vi "main.vi"() -> ()   [LabVIEW 2016]
uses:
  System Status.ctl
  Position Control.ctl
  Manual Operation Control.ctl
  Position Coordinate.ctl
panel:
  out "status":bool
  in  "Test Mode":bool
  in  "Leave HWLS":bool
  in  "Reference":bool
  in  "Reset Motion":bool
  in  "Stop Motion":bool
  in  "Manual Operation Control":T1 {"Speed Override (%)" min=0.0 max=150.0 step=1.0 scale=0.0..150.0; "Rotative"."Step Length" min=0.01 max=100.0 step=0.01; "Rotative"."Speed" min=0.0 max=500.0 step=1.0 scale=0.0..500.0 scale format="%#.0f"; "Linear"."Step Length" min=0.01 max=500.0 step=0.01; "Linear"."Speed" min=0.0 max=500.0 step=1.0 scale=0.0..500.0 scale format="%#.0f"}
  in  "Settings":bool
  in  "Exit":bool
  in  "Initialize":bool
  in  "Auto Run":bool
  in  "Auto Run Control":T2[](array[typedef])
  in  "Rel Position":T3={"Pos X"=0.0, "Position Name"="Rel Move", "Pos Y"=0.0, "Pos Z"=0.0, "Pos A"=0.0, "OK Button"=FALSE, "Normal Move"=FALSE, "Fast Move"=FALSE} {"Pos A" format="%.2f"; "Pos Z" format="%.2f"; "Pos Y" format="%.2f"; "Pos X" format="%.2f"}
  in  "Abs Position":T3={"Pos X"=0.0, "Position Name"="Abs Move", "Pos Y"=0.0, "Pos Z"=0.0, "Pos A"=0.0, "OK Button"=FALSE, "Normal Move"=FALSE, "Fast Move"=FALSE} {"Pos A" format="%.2f"; "Pos Z" format="%.2f"; "Pos Y" format="%.2f"; "Pos X" format="%.2f"}
  out "System Status":T4 {"Axis A"."Position" format="%.2f"; "Axis Z"."Position" format="%.2f"; "Axis Y"."Position" format="%.2f"; "Rotativ Speed" format="%#_6f"; "Linear Speed" format="%#.2f"; "Axis X"."Position" format="%.2f"}
  out "Error Information":string
  in  "MotionLibrary Path":path=path "C:/Program Files (x86)/National Instruments/LabVIEW 2016/user.lib/iselmotion/CNCAPI/CtrlDll/Dummy/mctlDummy.dll"
  out "Motor hModule":i32
  in  "MotionIni File In":path=path "C:/Program Files (x86)/National Instruments/LabVIEW 2016/user.lib/iselmotion/CNCAPI/CtrlDll/Dummy/MctlDummy.INI"
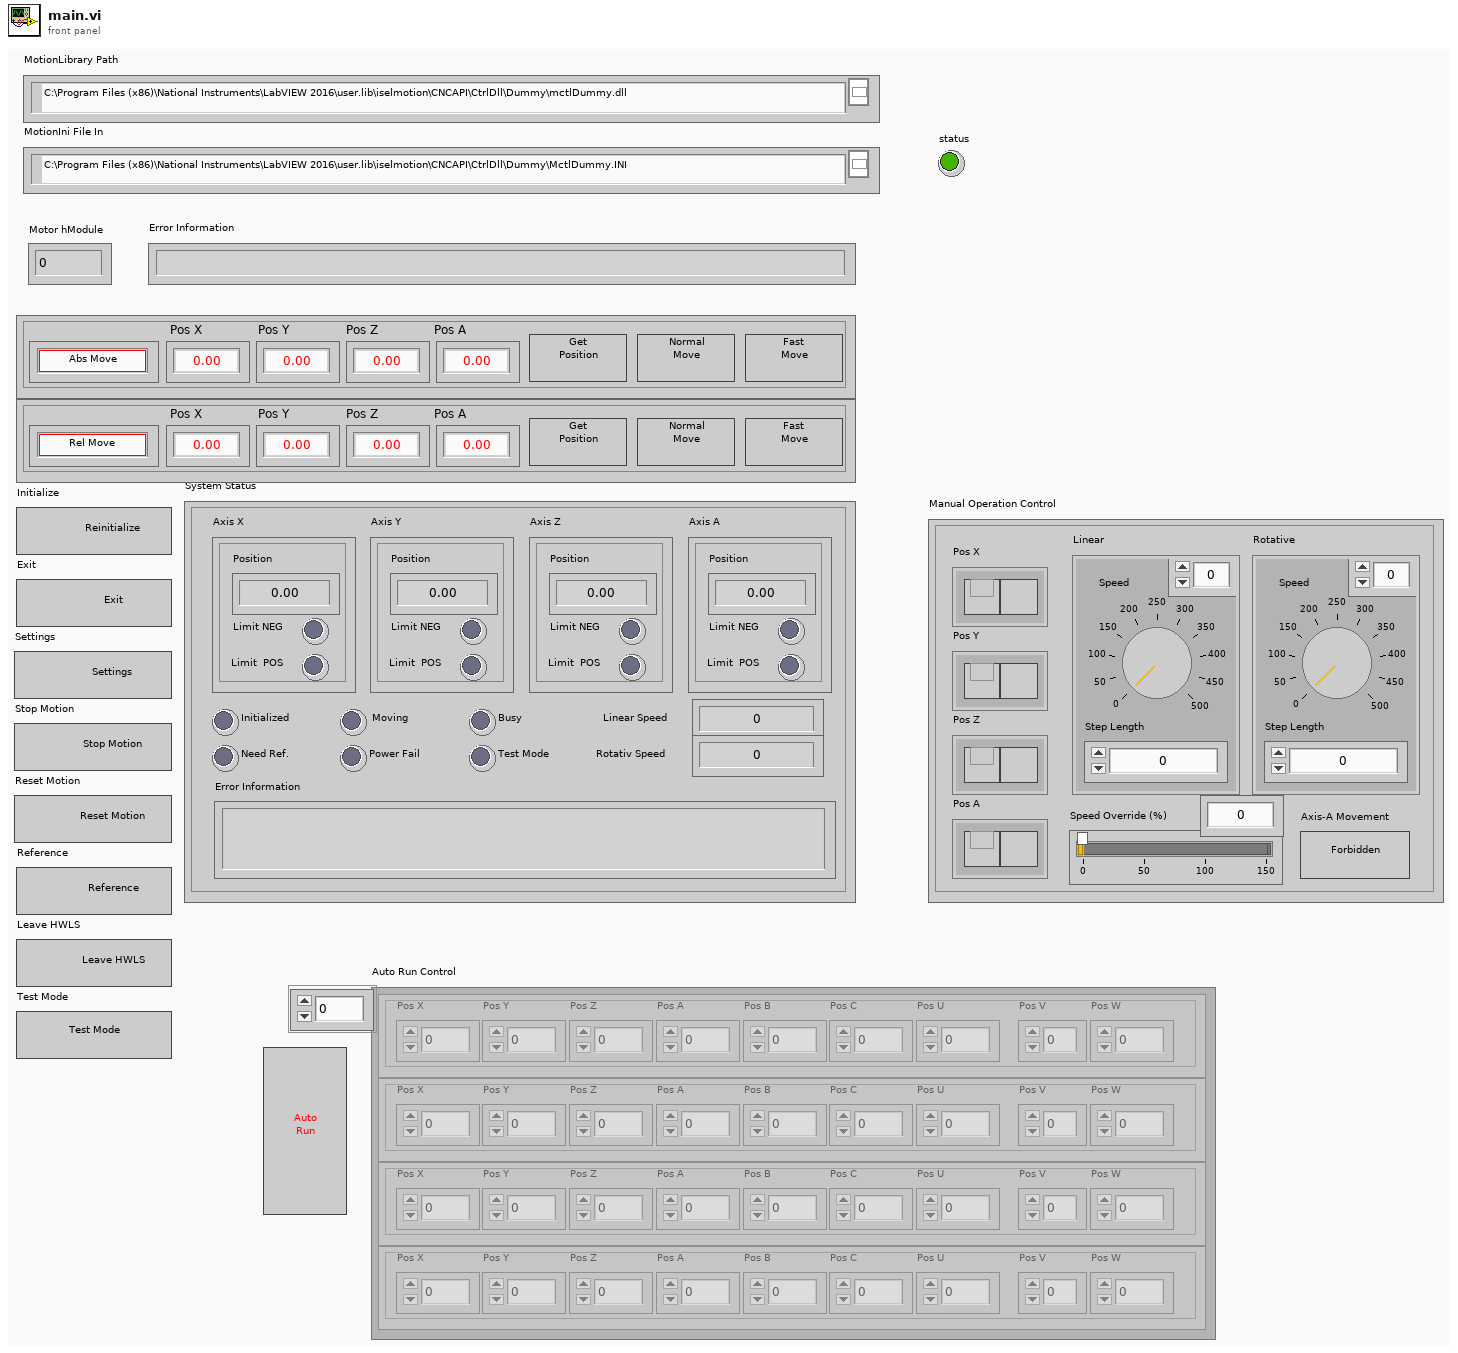
[diagram p1: front panel]
types:
  T1 = typedef "Manual Operation Control.ctl" = cluster{"Pos X":cluster{"Plus":bool, "Minus":bool}, "Pos Y":cluster{"Plus":bool, "Minus":bool}, "Pos Z":cluster{"Plus":bool, "Minus":bool}, "Pos A":cluster{"Plus":bool, "Minus":bool}, "Linear":cluster{"Speed":dbl, "Step Length":dbl}, "Rotative":cluster{"Speed":dbl, "Step Length":dbl}, "Speed Override (%)":dbl, "Axis-A Movement":bool}
  T2 = typedef "Position Coordinate.ctl" = cluster{"Pos X":dbl, "Pos Y":dbl, "Pos Z":dbl, "Pos A":dbl, "Pos B":dbl, "Pos C":dbl, "Pos U":dbl, "Pos V":dbl, "Pos W":dbl}
  T3 = typedef "Position Control.ctl" = cluster{"Pos X":dbl, "Position Name":string, "Pos Y":dbl, "Pos Z":dbl, "Pos A":dbl, "OK Button":bool, "Normal Move":bool, "Fast Move":bool}
  T4 = typedef "System Status.ctl" = cluster{"Axis X":cluster{"Position":dbl, "Limit NEG":bool, "Limit  POS":bool}, "Axis Y":cluster{"Position":dbl, "Limit NEG":bool, "Limit  POS":bool}, "Axis Z":cluster{"Position":dbl, "Limit NEG":bool, "Limit  POS":bool}, "Axis A":cluster{"Position":dbl, "Limit NEG":bool, "Limit  POS":bool}, "Initialized":bool, " Moving":bool, "Busy":bool, "Need Ref.":bool, "Power Fail":bool, "Test Mode":bool, "Linear Speed":dbl, "Rotativ Speed":dbl, "Error Information":string}
  T5 = enum16{"open", "replace", "create", "open or create", "replace or create", "replace or create with confirmation"}
  T6 = enum8{"Enabled", "Disabled", "Disabled and Grayed Out"}
  T7 = cluster{"PosX":i32, "PosY":i32, "PosZ":i32, "PosA":i32, "PosB":i32, "PosC":i32, "PosU":i32, "PosV":i32, "PosW":i32}
  T8 = cluster{"MotionLibrary Path":path, "MotionIni File In":path}
  T9 = cluster{"Common":cluster{"INMOTION":bool, "INSTOPMODE":bool, "INTEACHMODE":bool, "INTESTMODE":bool, "CURRENTOFF":bool, "INPATHMOTION":bool, "ISMOVING":bool, "PATHSTARTED":bool, "NEEDREFERENCERUN":bool, "BREAKERROR":bool, "HWLSACTIVE":bool, "SWLSACTIVE":bool, "HWLSDURINGMOTION":bool, "AFTERRUNERROR":bool, "LOADPATHDATAERROR":bool, "KEYSWITCHERROR":bool, "KEYSWDURINGMOTION":bool, "POWER_FAIL":bool, "SC_FAIL":bool, "HARDWARE_FAIL":bool, "COMMUNICATION_FAIL":bool}, "HWLSNeg":cluster{"HWLS_X_NEG":bool, "HWLS_Y_NEG":bool, "HWLS_Z_NEG":bool, "HWLS_A_NEG":bool, "HWLS_B_NEG":bool, "HWLS_C_NEG":bool, "HWLS_U_NEG":bool, "HWLS_V_NEG":bool, "HWLS_W_NEG":bool}, "HWLSPos":cluster{"HWLS_X_POS":bool, "HWLS_Y_POS":bool, "HWLS_Z_POS":bool, "HWLS_A_POS":bool, "HWLS_B_POS":bool, "HWLS_C_POS":bool, "HWLS_U_POS":bool, "HWLS_V_POS":bool, "HWLS_W_POS":bool}, "SWLSNeg":cluster{"SWLS_X_NEG":bool, "SWLS_Y_NEG":bool, "SWLS_Z_NEG":bool, "SWLS_A_NEG":bool, "SWLS_B_NEG":bool, "SWLS_C_NEG":bool, "SWLS_U_NEG":bool, "SWLS_V_NEG":bool, "SWLS_W_NEG":bool}, "SWLSPos":cluster{"SWLS_X_POS":bool, "SWLS_Y_POS":bool, "SWLS_Z_POS":bool, "SWLS_A_POS":bool, "SWLS_B_POS":bool, "SWLS_C_POS":bool, "SWLS_U_POS":bool, "SWLS_V_POS":bool, "SWLS_W_POS":bool}, "Extended":cluster{"ISBUSY":bool, "DISABLED":bool, "ISINITIALIZED":bool, "READY":bool, "DRILLCYCLEACTIVE":bool, "CTRLSPECERROR":bool}, "Additional flags":cluster{"InMotion":bool, "InStopMode":bool, "InTeachMode":bool, "InTestMode":bool, "CurrentOff":bool, "InPathMotion":bool, "IsMoving":bool, "NeedReferenceRun":bool, "BreakError":bool, "HWLSActive":bool, "SWLSActive":bool, "HWLSDuringMotion":bool, "AfterRunError":bool, "PowerFail":bool, "SCFail":bool, "IsBusy":bool, "Initialized":bool, "Disabled":bool, "HardwareFail":bool, "CommunicationFail":bool, "DrillCycleActive":bool, "CtrlSpecError":bool, "PathStarted":bool}}
  T10 = cluster{"PosX":dbl, "PosY":dbl, "PosZ":dbl, "PosA":dbl, "PosB":dbl, "PosC":dbl, "PosU":dbl, "PosV":dbl, "PosW":dbl}
  T11 = cluster{"PosX":dbl, "HWLS_X_NEG":bool, "HWLS_X_POS":bool}
  T12 = cluster{"PosY":dbl, "HWLS_Y_NEG":bool, "HWLS_Y_POS":bool}
  T13 = cluster{"PosZ":dbl, "HWLS_Z_NEG":bool, "HWLS_Z_POS":bool}
  T14 = cluster{dbl, "HWLS_A_NEG":bool, "HWLS_A_POS":bool}
  T15 = cluster{"LiNormVel":i32, "DrNormVel":i32, "LiFastVel":i32, "DrFastVel":i32, "LiTeachVel":i32, "DrTeachVel":i32, "LiActVel":i32, "DrActVel":i32}
  T16 = cluster{"LiNormVel":dbl, "DrNormVel":dbl, "LiFastVel":dbl, "DrFastVel":dbl, "LiTeachVel":dbl, "DrTeachVel":dbl, "LiActVel":dbl, "DrActVel":dbl}
  T17 = cluster{"Ability":cluster{"LINEAR":bool, "CIRCLE":bool, "HELIX":bool, "SPLINE":bool, "BEZIER":bool, "PRECALC":bool, "ONLINE":bool}, "NumAxis":u32, "AxisConfig":cluster{"AxisConfig 0":cluster{"Type":cluster{"LINEAR":bool, "ROT":bool}, "In Use":bool, "ID":u32, "RangeMin":u32, "RangeMax":u32}, "AxisConfig 1":cluster{"Type":cluster{"LINEAR":bool, "ROT":bool}, "In Use":bool, "ID":u32, "RangeMin":u32, "RangeMax":u32}, "AxisConfig 2":cluster{"Type":cluster{"LINEAR":bool, "ROT":bool}, "In Use":bool, "ID":u32, "RangeMin":u32, "RangeMax":u32}, "AxisConfig 3":cluster{"Type":cluster{"LINEAR":bool, "ROT":bool}, "In Use":bool, "ID":u32, "RangeMin":u32, "RangeMax":u32}, "AxisConfig 4":cluster{"Type":cluster{"LINEAR":bool, "ROT":bool}, "In Use":bool, "ID":u32, "RangeMin":u32, "RangeMax":u32}, "AxisConfig 5":cluster{"Type":cluster{"LINEAR":bool, "ROT":bool}, "In Use":bool, "ID":u32, "RangeMin":u32, "RangeMax":u32}, "AxisConfig 6":cluster{"Type":cluster{"LINEAR":bool, "ROT":bool}, "In Use":bool, "ID":u32, "RangeMin":u32, "RangeMax":u32}, "AxisConfig 7":cluster{"Type":cluster{"LINEAR":bool, "ROT":bool}, "In Use":bool, "ID":u32, "RangeMin":u32, "RangeMax":u32}, "AxisConfig 8":cluster{"Type":cluster{"LINEAR":bool, "ROT":bool}, "In Use":bool, "ID":u32, "RangeMin":u32, "RangeMax":u32}}}
  T18 = cluster{"In Use":bool, "In Use":bool, "In Use":bool, "In Use":bool, "In Use":bool, "In Use":bool, "In Use":bool, "In Use":bool, "In Use":bool}
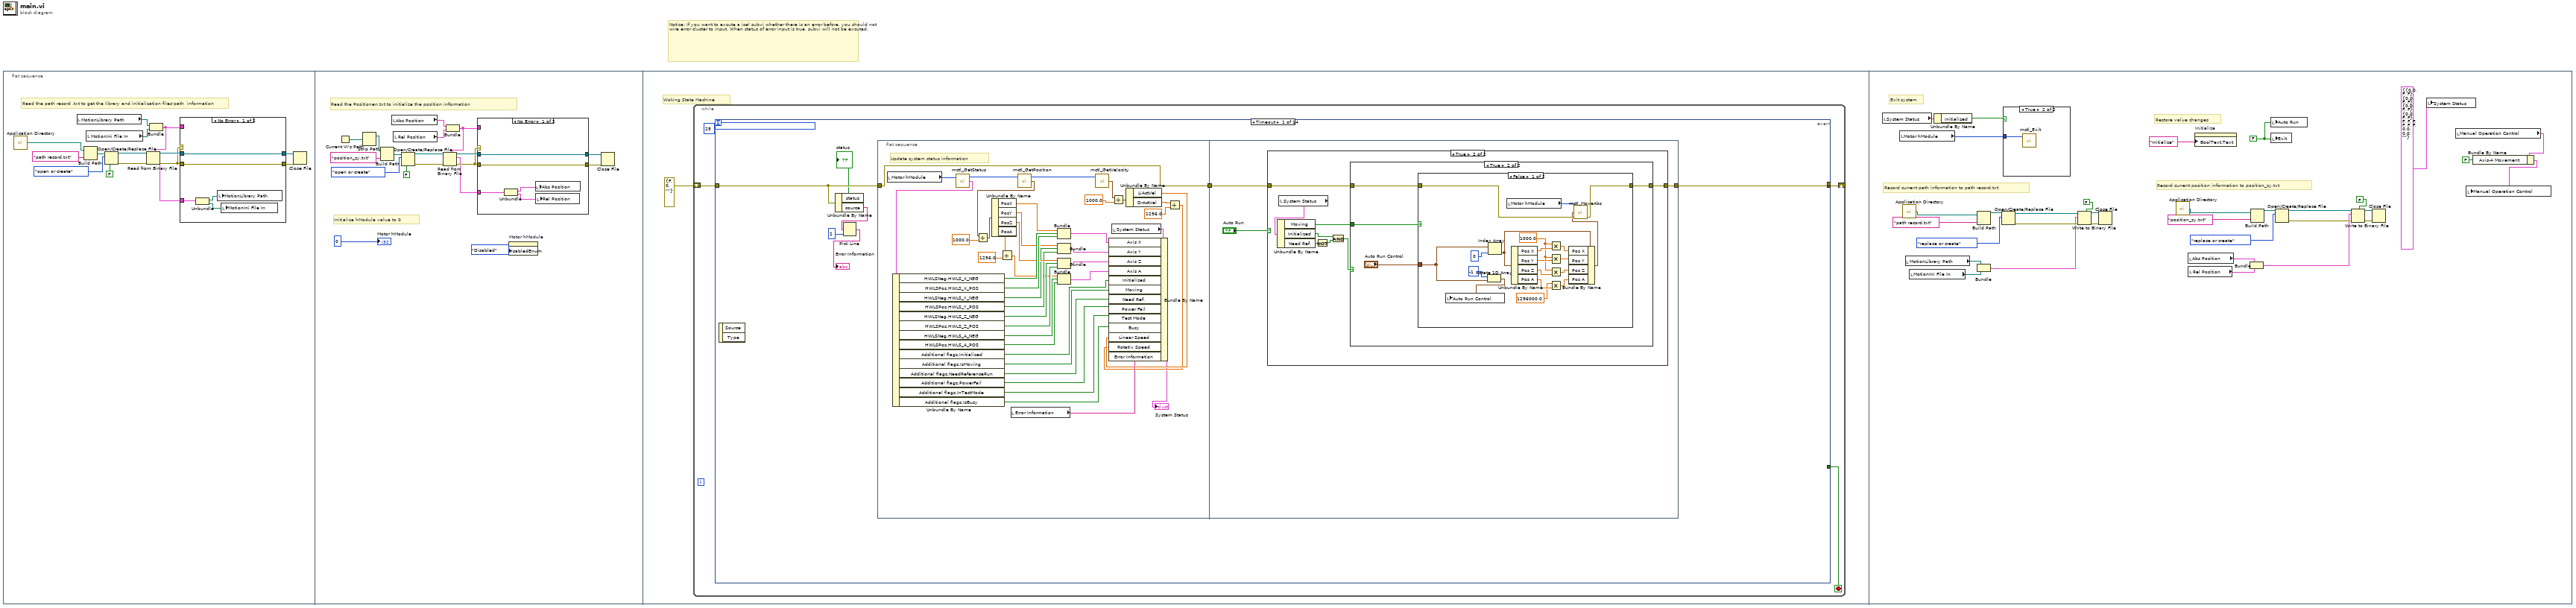
[diagram p0: block diagram]
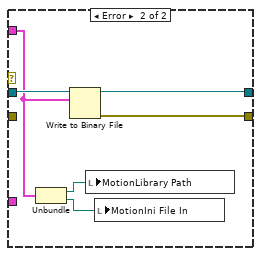
[diagram p2: hidden frame]
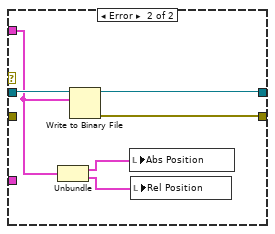
[diagram p3: hidden frame]
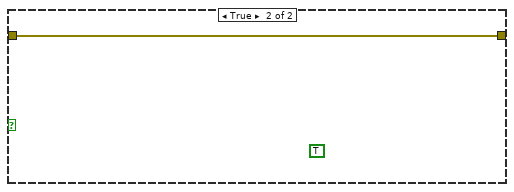
[diagram p6: hidden frame]
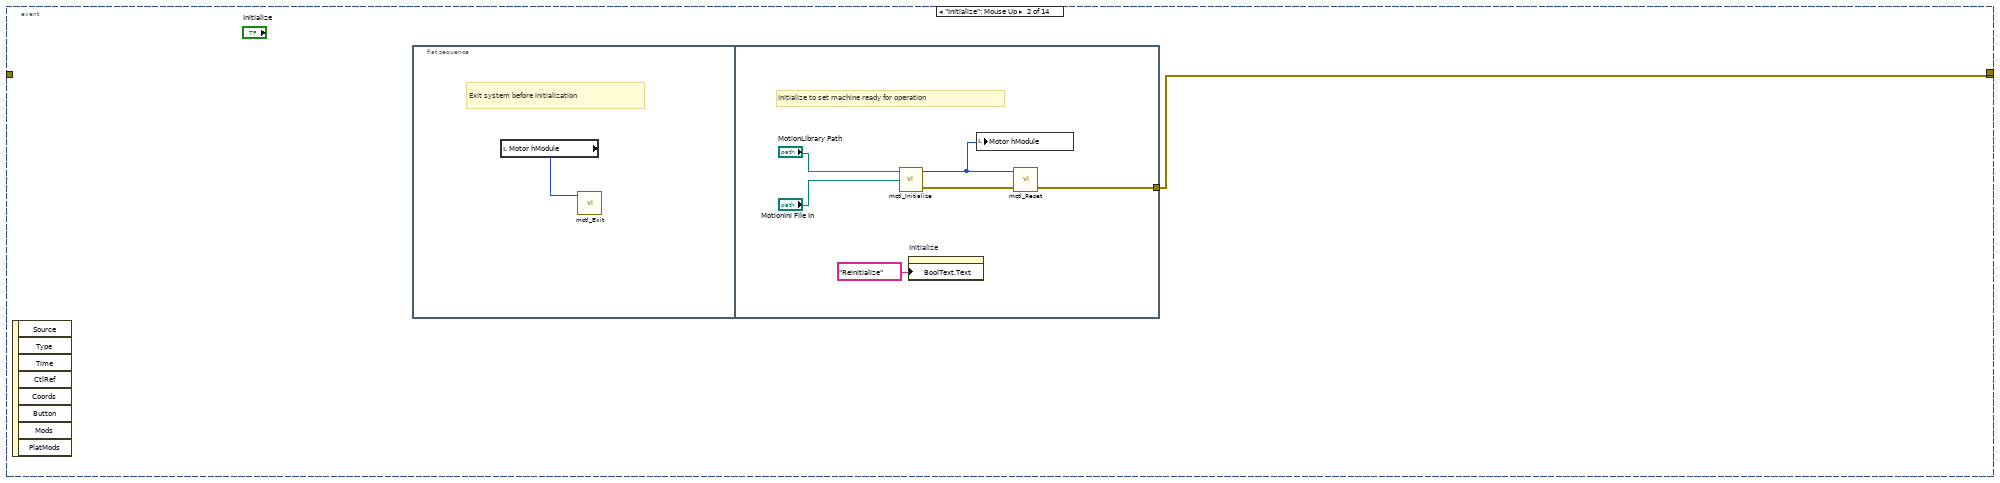
[diagram p7: hidden frame]
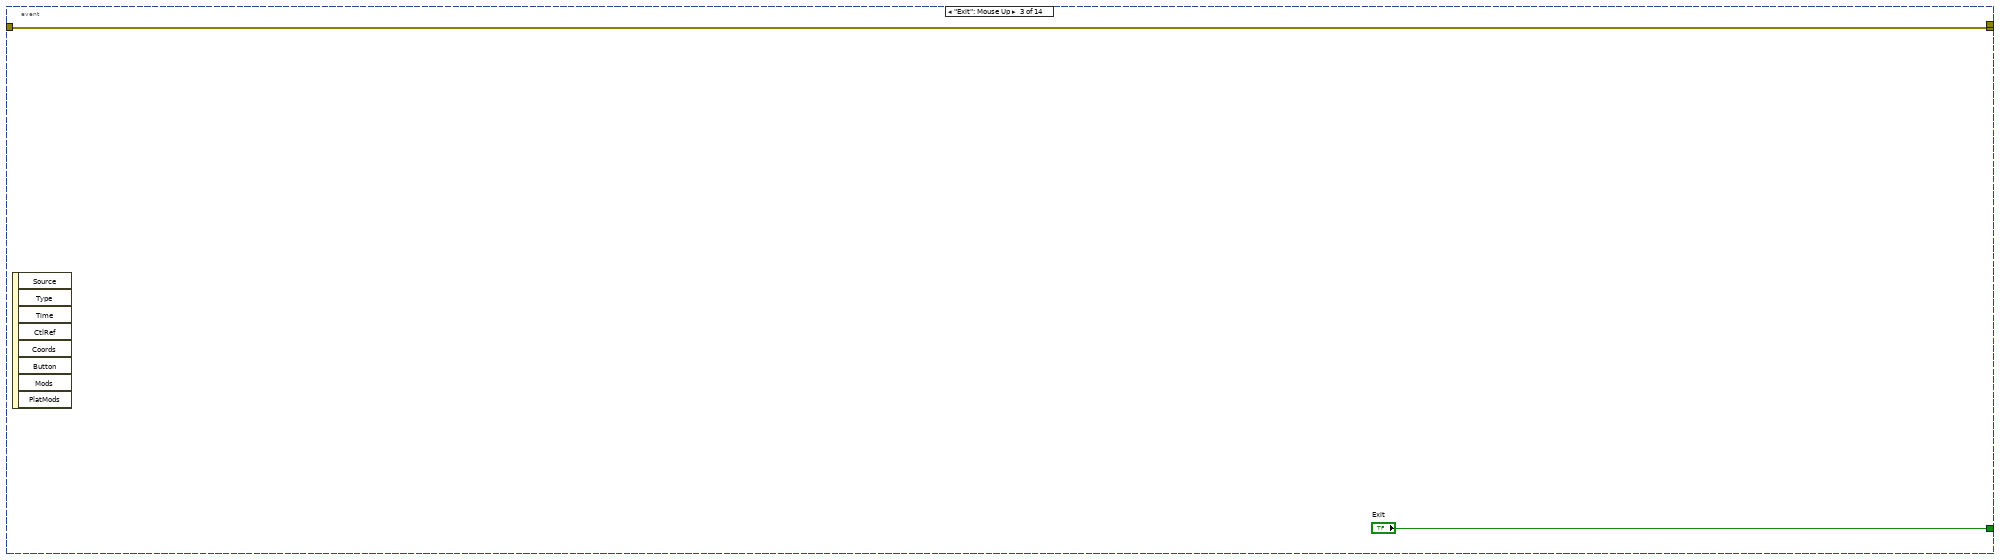
[diagram p8: hidden frame]
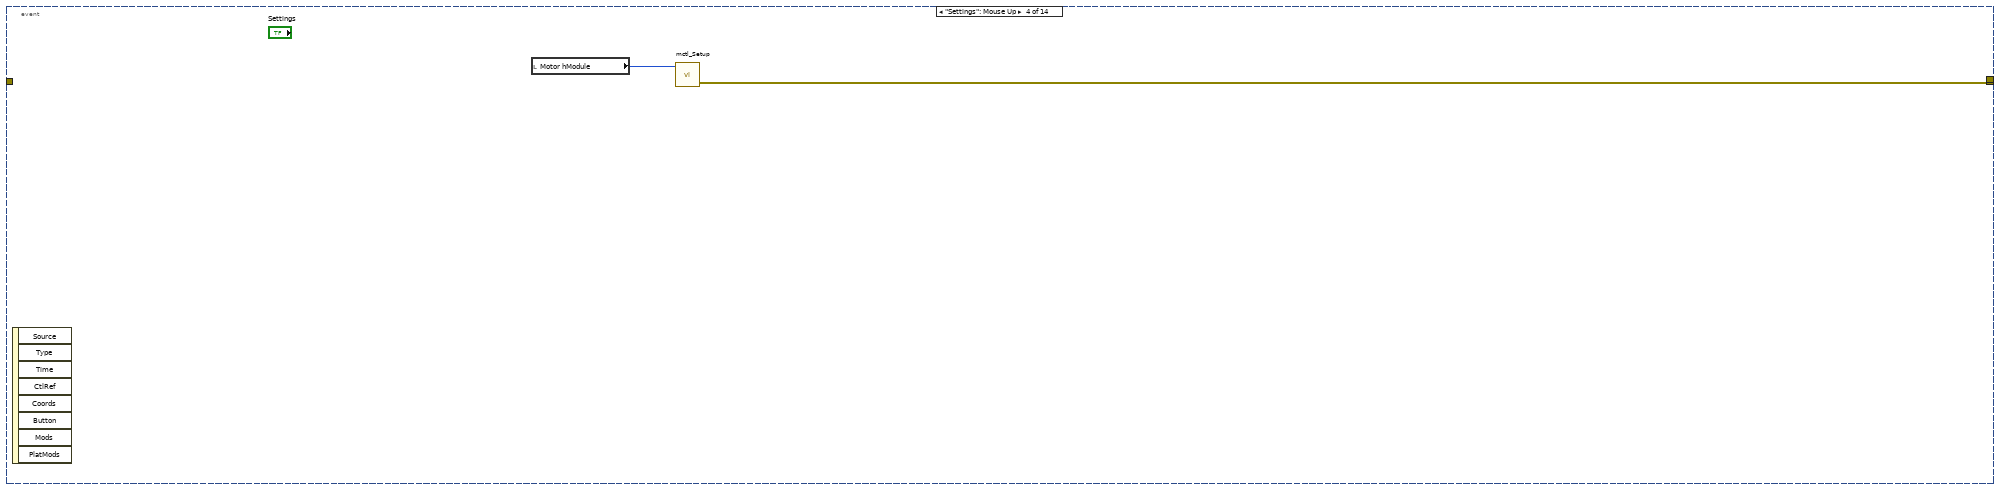
[diagram p9: hidden frame]
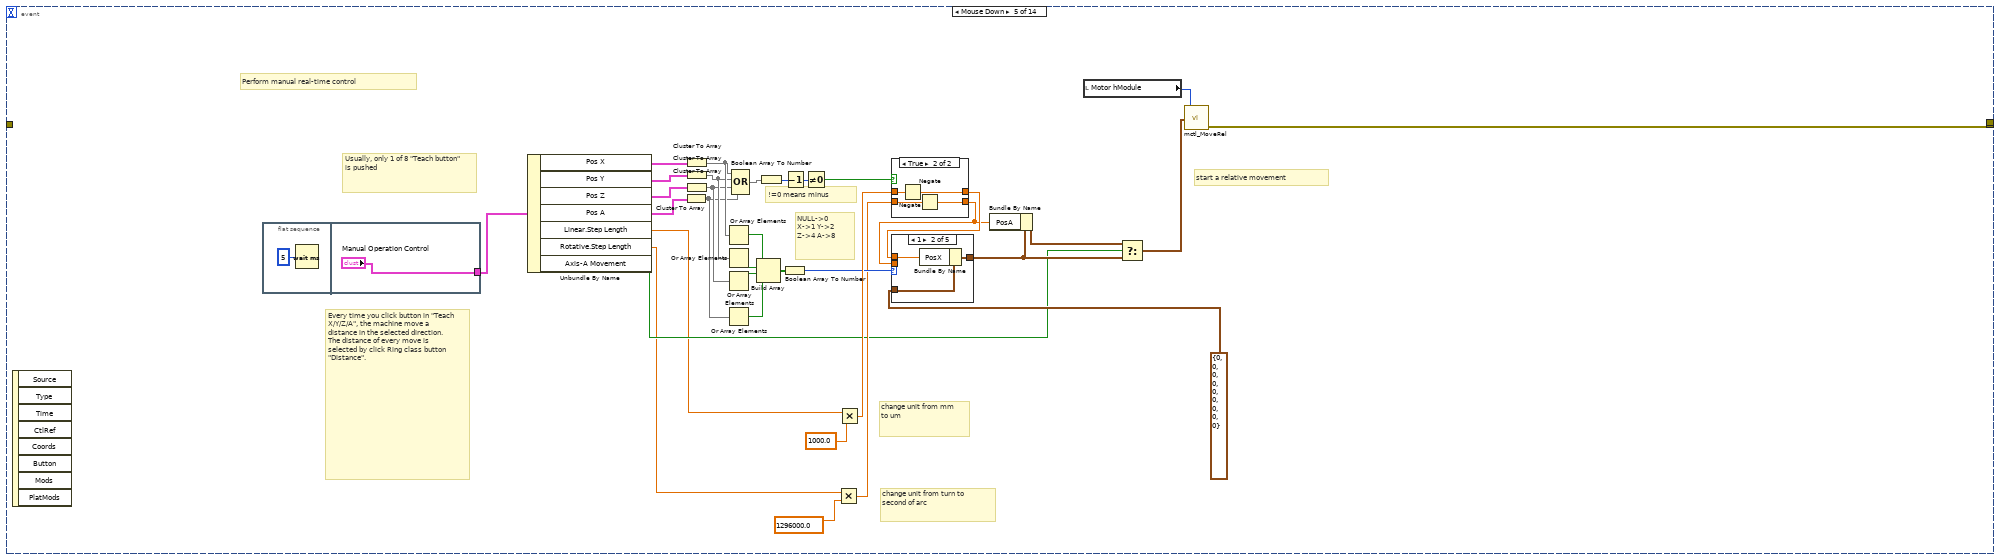
[diagram p10: hidden frame]
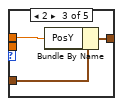
[diagram p12: hidden frame]
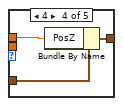
[diagram p13: hidden frame]
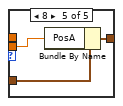
[diagram p14: hidden frame]
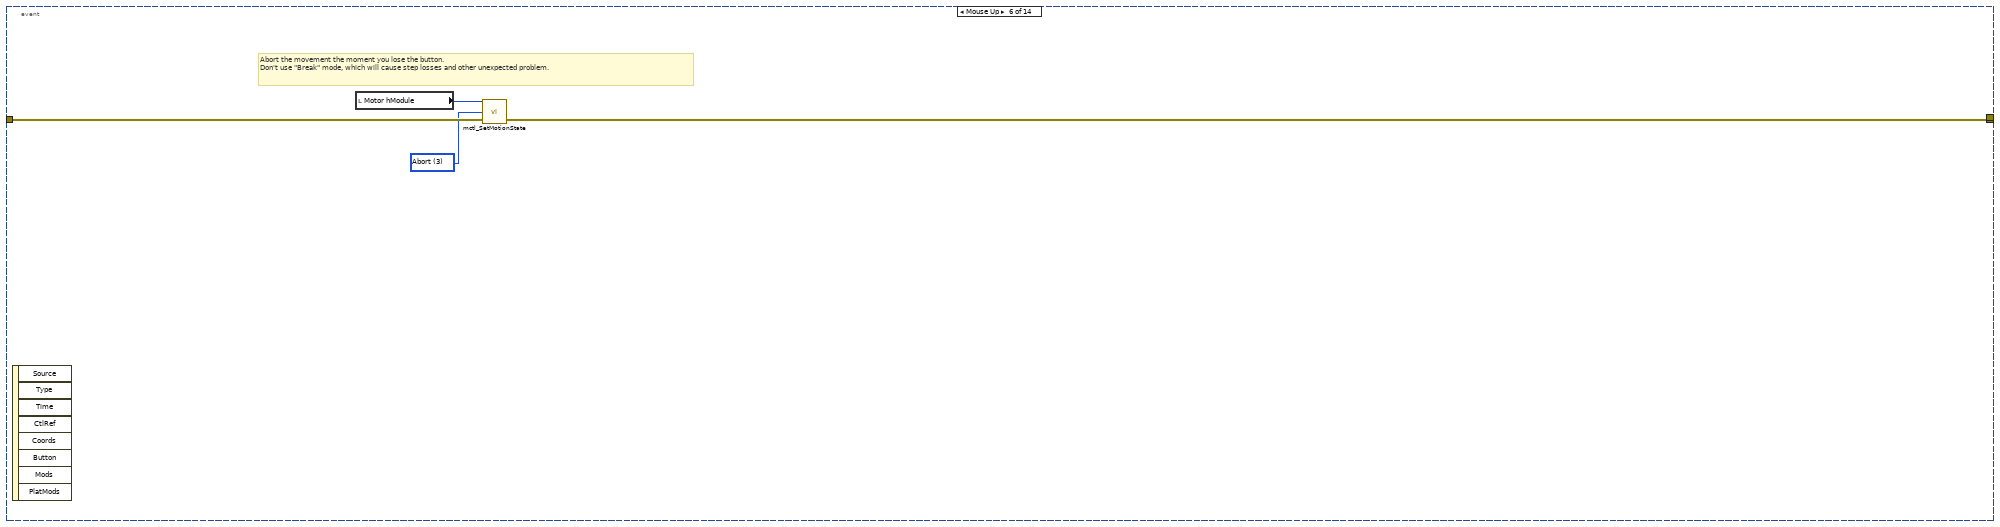
[diagram p16: hidden frame]
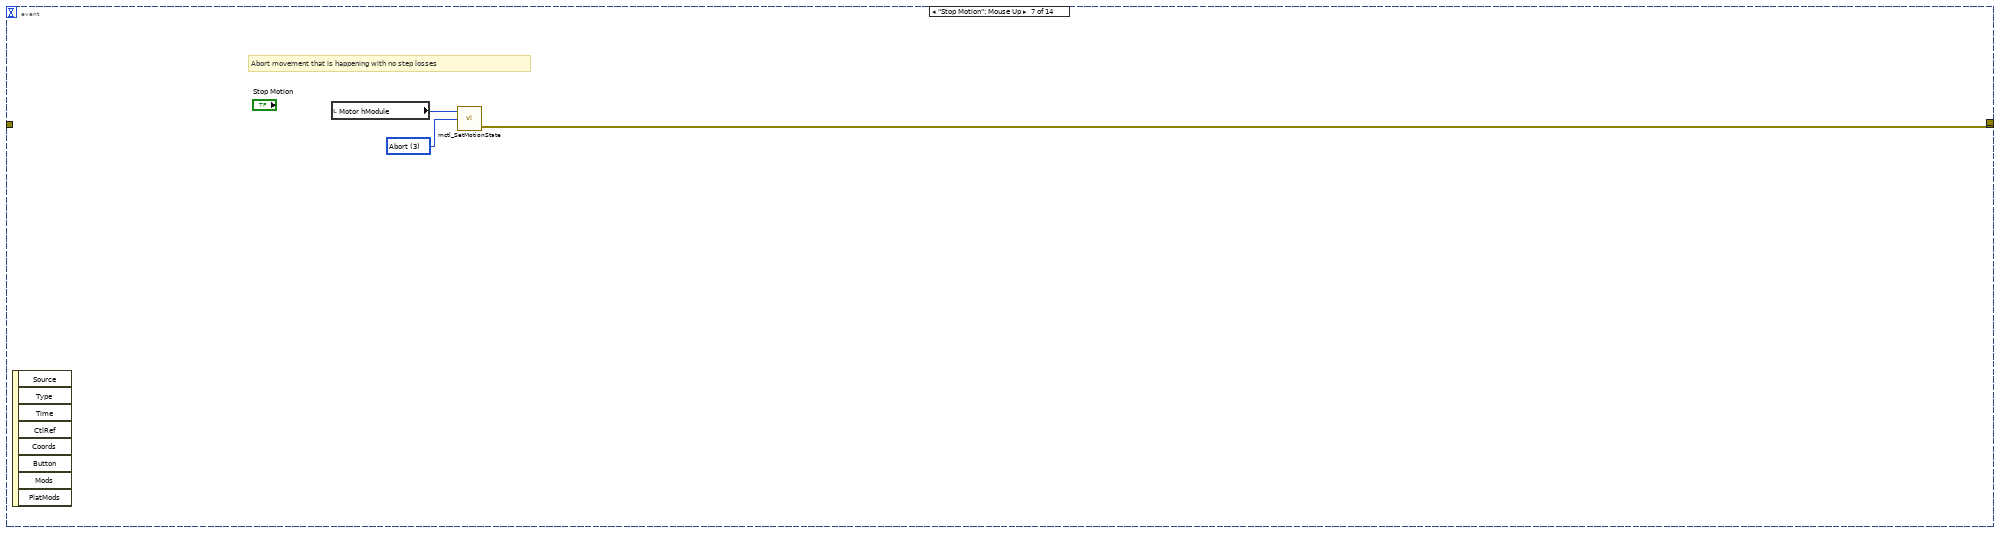
[diagram p17: hidden frame]
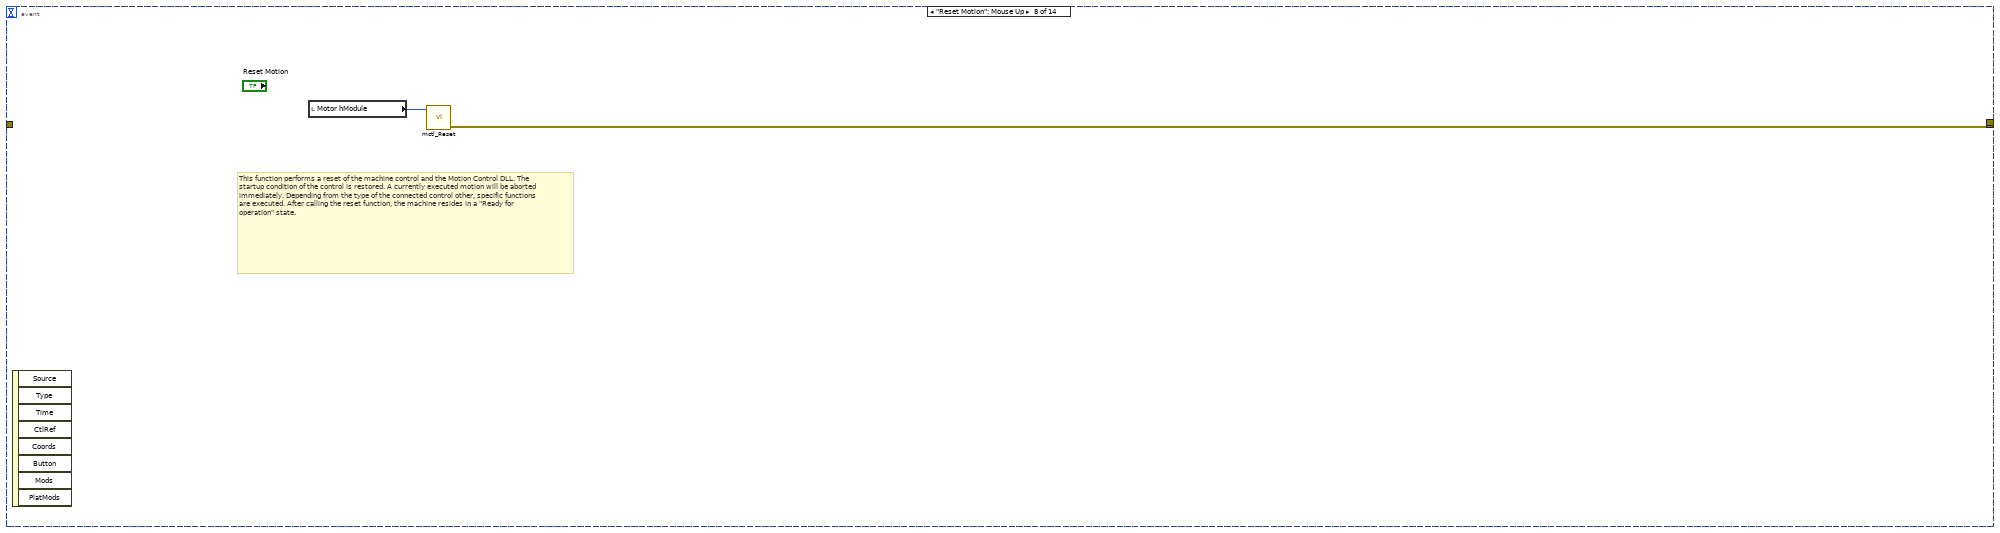
[diagram p18: hidden frame]
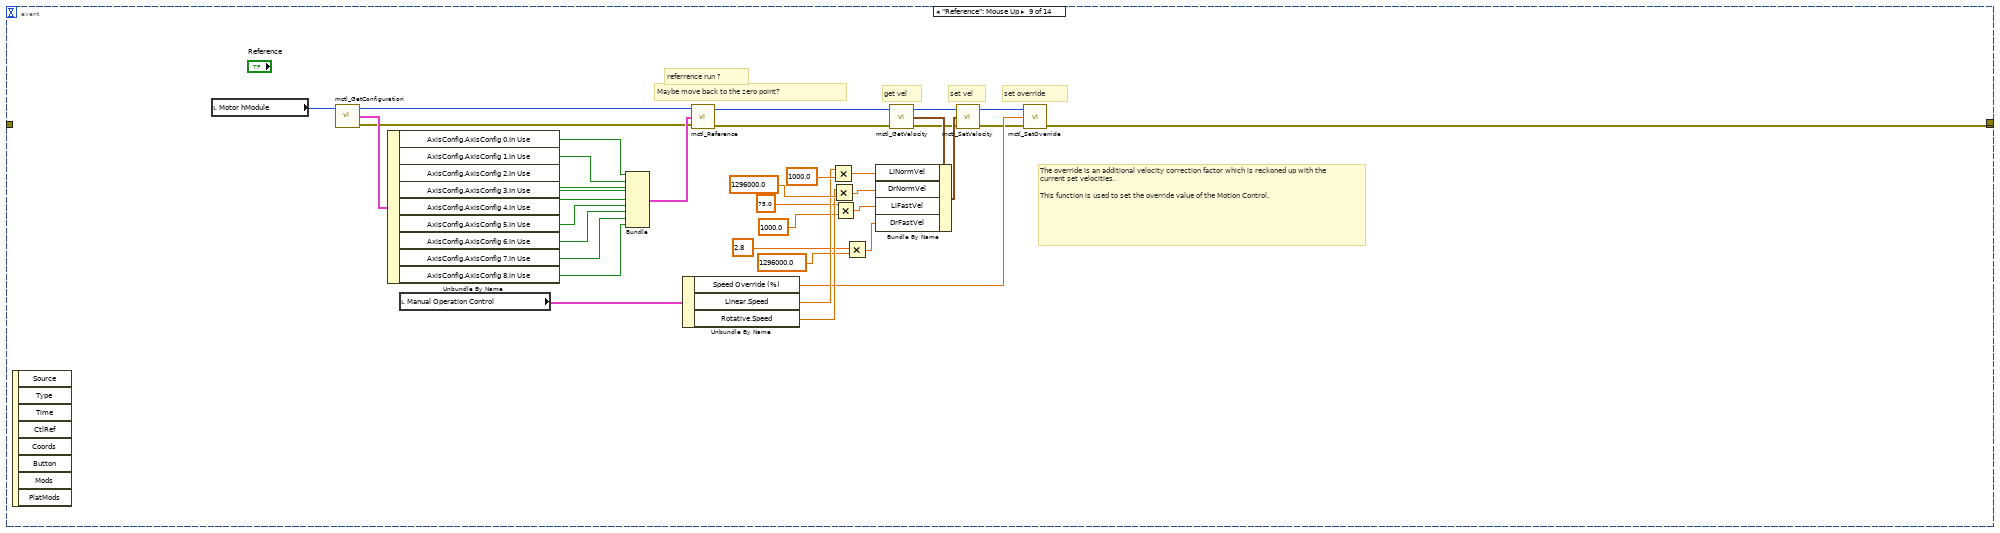
[diagram p19: hidden frame]
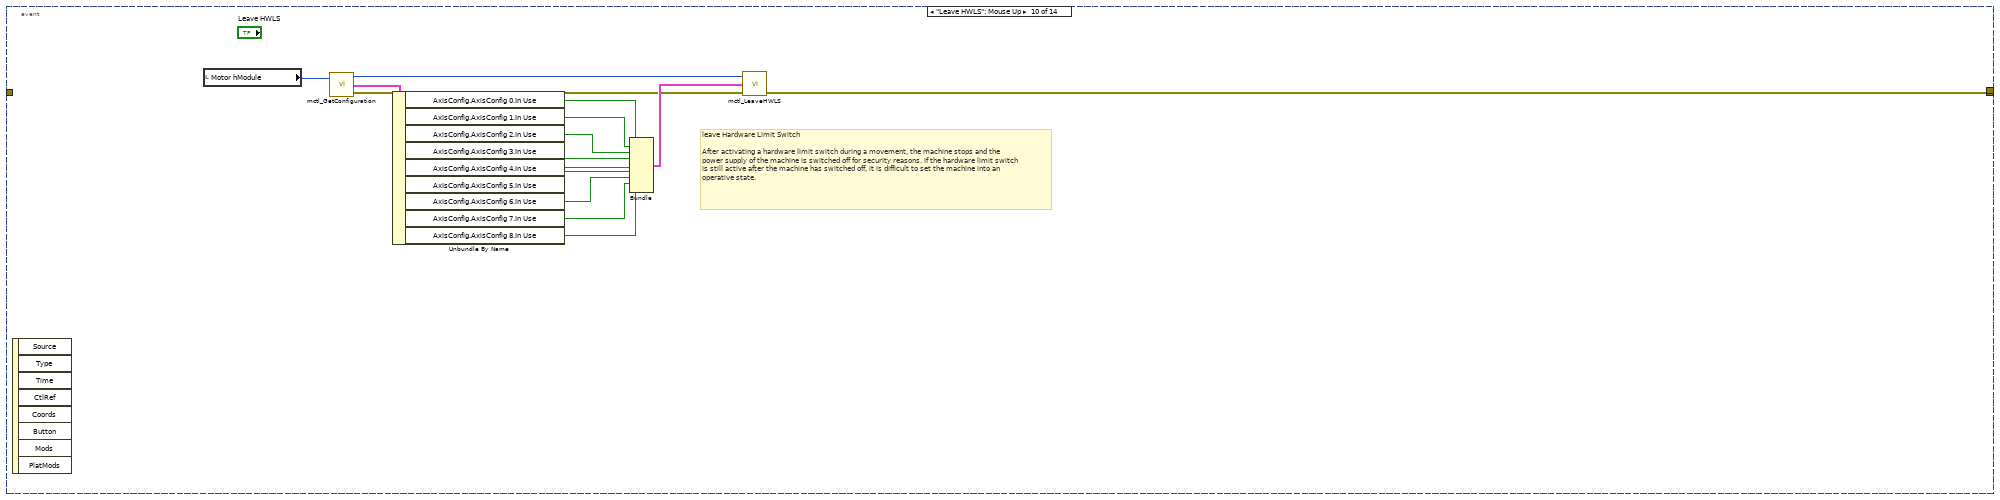
[diagram p20: hidden frame]
diagram:
  # "Notice: If you want to excute a isel subvi whether there is an error before, you should not wire error cluster to input. When status of error input is true, subvi will not be excuted."
  n1 = flat-sequence {
    frame #0 {
      # "Read the path record .txt to get the library and initialization files'path  information"
      n2 = call <vilib>:"Application Directory.vi"() -> ("Application Directory"=w2:path)
      n3 = local read "MotionLibrary Path"() -> (w10:path)
      n4 = Build Path(base path=w2, name or relative path="path record.txt") -> (appended path=w13:path)
      n5 = local read "MotionIni File In"() -> (w11:path)
      n6 = Open/Create/Replace File(file path (use dialog)=w13, operation (0:open)=T5."open or create", disable buffering (F)=FALSE ("advisory dialog? (display:T)")) -> (refnum out=w15:refnum<file>, error out=w12:errorcluster)  [unwired: 3 in, 1 out]
      n7 = Bundle("MotionLibrary Path"=w10, "MotionIni File In"=w11) -> (w3:T8)  [unwired: 1 in]
      n8 = Read from Binary File(5:w3, 8:w12, 11:w15) -> (0:w4:errorcluster, 2:w1:T8, 3:w7:refnum<file>)  [unwired: 3 in, 1 out]
      n9 = case shown="No Error" w4 {
        tunnel: w7 -> [w20 w26]
        tunnel: [w20 w24] -> w6
        tunnel: [w19 w25] -> w5
        tunnel: w4 -> [w19 _]
        tunnel: w3 -> [_ w23]
        tunnel: w1 -> [w18 _]
        frame No Error {
          n10 = Unbundle(w18) -> ("MotionLibrary Path"=w17:path, "MotionIni File In"=w16:path)
          n11 = local write "MotionLibrary Path"(w17) -> ()
          n12 = local write "MotionIni File In"(w16) -> ()
        }
        frame Error {
          n13 = Unbundle(w23) -> ("MotionLibrary Path"=w22:path, "MotionIni File In"=w21:path)
          n14 = Write to Binary File(file (use dialog)=w26, data=w23) -> (refnum out=w24:refnum<file>, error out=w25:errorcluster)  [unwired: 4 in, 1 out]
          n15 = local write "MotionLibrary Path"(w22) -> ()
          n16 = local write "MotionIni File In"(w21) -> ()
        }
      }
      n17 = Close File(refnum=w6, error in=w5) -> ()  [unwired: 2 out]
    }
    frame #1 {
      # "Initialize hModule value to 0"
      # "Read the Positionen.txt to initialize the position information"
      n18 = Current VI's Path() -> (path=w30:path)
      n19 = Strip Path(path=w30) -> (stripped path=w43:path)  [unwired: 1 out]
      n20 = Build Path(base path=w43, name or relative path="position_zy.txt") -> (appended path=w41:path)
      n21 = local read "Abs Position"() -> (w38:T3)
      n22 = local read "Rel Position"() -> (w39:T3)
      n23 = Open/Create/Replace File(file path (use dialog)=w41, operation (0:open)=T5."open or create", disable buffering (F)=FALSE ("advisory dialog? (display:T)")) -> (refnum out=w44:refnum<file>, error out=w40:errorcluster)  [unwired: 3 in, 1 out]
      n24 = Bundle("Abs Position"=w38, "Rel Position"=w39) -> (w31:cluster{"Abs Position":T3, "Rel Position":T3})  [unwired: 1 in]
      n25 = Read from Binary File(5:w31, 8:w40, 11:w44) -> (0:w32:errorcluster, 2:w28:cluster{"Abs Position":T3, "Rel Position":T3}, 3:w35:refnum<file>)  [unwired: 3 in, 1 out]
      n26 = case shown="No Error" w32 {
        tunnel: w35 -> [w49 w55]
        tunnel: [w49 w53] -> w34
        tunnel: [w48 w54] -> w33
        tunnel: w32 -> [w48 _]
        tunnel: w31 -> [_ w52]
        tunnel: w28 -> [w47 _]
        frame No Error {
          n27 = Unbundle(w47) -> ("Abs Position"=w46:T3, "Rel Position"=w45:T3)
          n28 = local write "Abs Position"(w46) -> ()
          n29 = local write "Rel Position"(w45) -> ()
        }
        frame Error {
          n30 = Unbundle(w52) -> ("Abs Position"=w51:T3, "Rel Position"=w50:T3)
          n31 = Write to Binary File(file (use dialog)=w55, data=w52) -> (refnum out=w53:refnum<file>, error out=w54:errorcluster)  [unwired: 4 in, 1 out]
          n32 = local write "Abs Position"(w51) -> ()
          n33 = local write "Rel Position"(w50) -> ()
        }
      }
      n34 = property on="Motor hModule" class="DigNum (strict)"("DisabledEnum"=T6."Disabled" ("Disabled")) -> ()  [unwired: 2 in, 2 out]
      n35 = Close File(refnum=w34, error in=w33) -> ()  [unwired: 2 out]
      "Motor hModule" <- 0
    }
    frame #2 {
      # "Woking State Machine"
      n36 = while {
        shift-right: [w58] -> _
        shift-left: errorcluster {"status"=FALSE, "code"=0, "source"=""} ("error constant") -> [w59]
        stop <- w57 stop-if-true
        n37 = event shown="[0] Timeout" {
          selector: _ -> [_ _ _ _ _ _ _ _ _ _ _ _ _ _]
          dyn-events: _ -> [_ _ _ _ _ _ _ _ _ _ _ _ _ _]
          timeout: 25 -> [_ _ _ _ _ _ _ _ _ _ _ _ _ _]
          tunnel: w59 -> [w67 _ w156 _ _ w218 _ _ _ _ _ w284 w334 _]
          tunnel: [w62 w148 w156 w158 w162 w217 w219 w222 w228 w267 w276 _ w333 w384] -> w58
          tunnel: [_ _ "Exit" _ _ _ _ _ _ _ _ _ _ _] -> w57
          tunnel: [_ _ _ _ _ _ _ _ _ _ _ w283 _ _] -> _
          event Timeout {
            n38 = event-data() -> ()  [unwired: 1 in, 2 out]
            n39 = Unbundle By Name(w67) -> ("status"=→"status":bool, "source"=w65:string)
            n40 = Pick Line(multi-line string=w65, line index=2) -> (output string=→"Error Information":string)  [unwired: 1 in]
            n41 = flat-sequence {
              tunnel: w67 -> [w69]
              tunnel: [w69] -> w63
              tunnel: w63 -> [w111]
              tunnel: [w110] -> w62
              frame #0 {
                # "Update system status information"
                n42 = local read "Motor hModule"() -> (w109:i32)
                n43 = call <userlib>:"mctl_GetStatus.vi"("hModule In"=w109) -> ("Status"=w108:T9, "hModule Out"=w107:u32)  [unwired: 2 in, 1 out]
                n44 = Unbundle By Name(w108) -> ("HWLSNeg.HWLS_X_NEG"=w101:bool, "HWLSPos.HWLS_X_POS"=w100:bool, "HWLSNeg.HWLS_Y_NEG"=w97:bool, "HWLSPos.HWLS_Y_POS"=w96:bool, "HWLSNeg.HWLS_Z_NEG"=w95:bool, "HWLSPos.HWLS_Z_POS"=w94:bool, "HWLSNeg.HWLS_A_NEG"=w93:bool, "HWLSPos.HWLS_A_POS"=w92:bool, "Additional flags.Initialized"=w87:bool, "Additional flags.IsMoving"=w86:bool, "Additional flags.NeedReferenceRun"=w85:bool, "Additional flags.PowerFail"=w82:bool, "Additional flags.InTestMode"=w83:bool, "Additional flags.IsBusy"=w84:bool)
                n45 = local read "Error Information"() -> (w81:string)
                n46 = call <userlib>:"mctl_GetPosition.vi"("hModule In"=w107) -> ("AxisPos"=w105:T7, "hModule Out"=w106:u32)  [unwired: 2 in, 1 out]
                n47 = Divide(x=w105, y=1000.0) -> (x/y=w103:T10)
                n48 = Unbundle By Name(w103) -> ("PosX"=w102:dbl, "PosY"=w99:dbl, "PosZ"=w98:dbl, "PosA"=w79:dbl)
                n49 = Divide(x=w79, y=1296.0) -> (x/y=w77:dbl)
                n50 = Bundle("PosX"=w102, "HWLS_X_NEG"=w101, "HWLS_X_POS"=w100) -> (w91:T11)  [unwired: 1 in]
                n51 = Bundle("PosY"=w99, "HWLS_Y_NEG"=w97, "HWLS_Y_POS"=w96) -> (w90:T12)  [unwired: 1 in]
                n52 = Bundle("PosZ"=w98, "HWLS_Z_NEG"=w95, "HWLS_Z_POS"=w94) -> (w89:T13)  [unwired: 1 in]
                n53 = Bundle(w77, "HWLS_A_NEG"=w93, "HWLS_A_POS"=w92) -> (w88:T14)  [unwired: 1 in]
                n54 = call <userlib>:"mctl_GetVelocity.vi"("hModule In"=w106) -> ("Velocity"=w74:T15)  [unwired: 2 in, 2 out]
                n55 = Divide(x=w74, y=1000.0) -> (x/y=w75:T16)
                n56 = local read "System Status"() -> (w80:T4)
                n57 = Unbundle By Name(w75) -> ("LiActVel"=w76:dbl, "DrActVel"=w72:dbl)
                n58 = Divide(x=w72, y=1296.0) -> (x/y=w70:dbl)
                n59 = Bundle By Name(cluster=w80, "Axis X"=w91, "Axis Y"=w90, "Axis Z"=w89, "Axis A"=w88, "Initialized"=w87, "Moving"=w86, "Need Ref."=w85, "Power Fail"=w82, "Test Mode"=w83, "Busy"=w84, "Linear Speed"=w76, "Rotativ Speed"=w70, "Error Information"=w81) -> (→"System Status":T4)
              }
              frame #1 {
                n60 = case shown="True" "Auto Run" {
                  tunnel: w111 -> [w113 w120]
                  tunnel: [w113 w119] -> w110
                  frame False {
                  }
                  frame True {
                    n61 = local read "System Status"() -> (w121:T4)
                    n62 = Unbundle By Name(w121) -> ("Moving"=w118:bool, "Initialized"=w116:bool, "Need Ref."=w117:bool)
                    n63 = Not(x=w117) -> (.not. x?=w114:bool)
                    n64 = And(x=w116, y=w114) -> (x .and. y?=w115:bool)
                    n65 = case shown="True" w115 {
                      tunnel: w120 -> [w122 w126]
                      tunnel: [w122 w123] -> w119
                      tunnel: w118 -> [_ w124]
                      frame False {
                      }
                      frame True {
                        n66 = case shown="False" w124 {
                          tunnel: w126 -> [w143 w147]
                          tunnel: [w140 w147] -> w123
                          tunnel: "Auto Run Control" -> [w141 _]
                          frame False {
                            w134 = 1000.0
                            n67 = Rotate 1D Array(1:w141, 2:-1 ("n")) -> (0:w139:T2[])
                            n68 = local write "Auto Run Control"(w139) -> ()
                            n69 = Index Array(array=w141, index=0) -> (element=w132:T2)
                            n70 = local read "Motor hModule"() -> (w142:i32)
                            n71 = Unbundle By Name(w132) -> ("Pos X"=w138:dbl, "Pos Y"=w137:dbl, "Pos Z"=w136:dbl, "Pos A"=w135:dbl)
                            n72 = Multiply(x=w134, y=w138) -> (x*y=w131:dbl)
                            n73 = Multiply(x=w134, y=w137) -> (x*y=w130:dbl)
                            n74 = Multiply(x=w134, y=w136) -> (x*y=w129:dbl)
                            n75 = Multiply(x=1296000.0, y=w135) -> (x*y=w128:dbl)
                            n76 = Bundle By Name(cluster=w132, "Pos X"=w131, "Pos Y"=w130, "Pos Z"=w129, "Pos A"=w128) -> (w127:T2)
                            n77 = call <userlib>:"mctl_MoveAbs.vi"("error in"=w143, "Abs"=w127, "hModule In"=w142) -> ("error out"=w140:errorcluster)  [unwired: 1 in, 1 out]
                          }
                          frame True {
                            w146 = TRUE
                          }
                        }
                      }
                    }
                  }
                }
              }
            }
          }
          event "Initialize": Mouse Up {
            n78 = event-data() -> ()  [unwired: 1 in, 8 out]
            n79 = flat-sequence {
              tunnel: [w154] -> w148
              frame #0 {
                # "Exit system before initialization"
                n80 = local read "Motor hModule"() -> (w149:i32)
                n81 = call <userlib>:"mctl_Exit.vi"("hModule In"=w149) -> ()  [unwired: 3 in, 2 out]
              }
              frame #1 {
                # "Initialize to set machine ready for operation"
                n82 = call <userlib>:"mctl_Initialize.vi"("Ini File In"="MotionIni File In", "Library In"="MotionLibrary Path") -> ("error out"=w155:errorcluster, "hModule Out"=w151:u32)  [unwired: 1 in, 1 out]
                n83 = property on="Initialize" class="Bool (strict)"("BoolText.Text"="Reinitialize" ("Boolean Text.Text")) -> ()  [unwired: 2 in, 2 out]
                n84 = local write "Motor hModule"(w151) -> ()
                n85 = call <userlib>:"mctl_Reset.vi"("error in"=w155, "hModule In"=w151) -> ("error out"=w154:errorcluster)  [unwired: 2 in, 1 out]
              }
            }
          }
          event "Exit": Mouse Up {
            n86 = event-data() -> ()  [unwired: 1 in, 8 out]
          }
          event "Settings": Mouse Up {
            n87 = event-data() -> ()  [unwired: 1 in, 8 out]
            n88 = local read "Motor hModule"() -> (w159:i32)
            n89 = call <userlib>:"mctl_Setup.vi"("hModule In"=w159) -> ("error out"=w158:errorcluster)  [unwired: 3 in, 1 out]
          }
          event Mouse Down {
            # "Usually, only 1 of 8 \"Teach button\" is pushed"
            # "!=0 means minus"
            # "change unit from turn to second of arc"
            # "change unit from mm to um"
            # "start a relative movement"
            # "Every time you click button in \"Teach X/Y/Z/A\", the machine move a distance in the selected direction. The distance of every move is selected by click Ring class button \"Distance\"."
            # "NULL->0\nX->1 Y->2\nZ->4 A->8"
            # "Perform manual real-time control"
            n90 = event-data() -> ()  [unwired: 1 in, 8 out]
            n91 = flat-sequence {
              tunnel: ["Manual Operation Control"] -> w165
              frame #0 {
                n92 = Wait (ms)(milliseconds to wait=u32 5) -> ()  [unwired: 1 out]
              }
              frame #1 {
              }
            }
            n93 = Unbundle By Name(w165) -> ("Pos X"=w193:cluster{"Plus":bool, "Minus":bool}, "Pos Y"=w192:cluster{"Plus":bool, "Minus":bool}, "Pos Z"=w191:cluster{"Plus":bool, "Minus":bool}, "Pos A"=w190:cluster{"Plus":bool, "Minus":bool}, "Linear.Step Length"=w161:dbl, "Rotative.Step Length"=w160:dbl, "Axis-A Movement"=w166:bool)
            n94 = Cluster To Array(cluster=w190) -> (array=w181:bool[])
            n95 = Cluster To Array(cluster=w193) -> (array=w184:bool[])
            n96 = Cluster To Array(cluster=w192) -> (array=w183:bool[])
            n97 = Cluster To Array(cluster=w191) -> (array=w182:bool[])
            n98 = Or Array Elements(Boolean array=w184) -> (logical OR=w189:bool)
            n99 = Or Array Elements(Boolean array=w183) -> (logical OR=w188:bool)
            n100 = Or Array Elements(Boolean array=w182) -> (logical OR=w187:bool)
            n101 = Or Array Elements(Boolean array=w181) -> (logical OR=w186:bool)
            n102 = Compound Arithmetic op=OR(w184, w183, w182, w181) -> (w178:bool[])
            n103 = Build Array(w189, w188, w187, w186) -> (w185:bool[])
            n104 = Boolean Array To Number(Boolean array=w178) -> (number=w180:u32)
            n105 = Boolean Array To Number(Boolean array=w185) -> (number=w175:u32)
            n106 = Decrement(x=w180) -> (x-1=w179:u32)
            n107 = Not Equal To 0?(x=w179) -> (x != 0?=w164:bool)
            n108 = Multiply(x=w160, y=1296000.0) -> (x*y=w171:dbl)
            n109 = Multiply(x=w161, y=1000.0) -> (x*y=w176:dbl)
            n110 = case shown="True" w164 {
              tunnel: w176 -> [w210 w214]
              tunnel: [w210 w213] -> w173
              tunnel: w171 -> [w209 w212]
              tunnel: [w209 w211] -> w169
              frame False {
              }
              frame True {
                n111 = Negate(x=w214) -> (-x=w213:dbl)
                n112 = Negate(x=w212) -> (-x=w211:dbl)
              }
            }
            n113 = case shown="1" w175 {
              tunnel: T7 {"PosX"=0, "PosY"=0, "PosZ"=0, "PosA"=0, "PosB"=0, "PosC"=0, "PosU"=0, "PosV"=0, "PosW"=0} ("RelPOS") -> [w196 w198 w201 w204 w207]
              tunnel: [w196 w199 w202 w205 w208] -> w170
              tunnel: w173 -> [_ w197 w200 w203 _]
              tunnel: w169 -> [_ _ _ _ w206]
              frame 0, Default {
              }
              frame 1 {
                n114 = Bundle By Name(cluster=w198, "PosX"=w197) -> (w199:T7)
              }
              frame 2 {
                n115 = Bundle By Name(cluster=w201, "PosY"=w200) -> (w202:T7)
              }
              frame 4 {
                n116 = Bundle By Name(cluster=w204, "PosZ"=w203) -> (w205:T7)
              }
              frame 8 {
                n117 = Bundle By Name(cluster=w207, "PosA"=w206) -> (w208:T7)
              }
            }
            n118 = Bundle By Name(cluster=w170, "PosA"=w169) -> (w168:T7)
            n119 = local read "Motor hModule"() -> (w163:i32)
            n120 = Select(t=w168, s=w166, f=w170) -> (s? t:f=w167:T7)
            n121 = call <userlib>:"mctl_MoveRel.vi"("RelPOS"=w167, "hModule In"=w163) -> ("error out"=w162:errorcluster)  [unwired: 2 in, 1 out]
          }
          event Mouse Up {
            w215 = u32 3 items=["Restart", "Stop", "Break", "Abort"] ("Motion State")
            # "Abort the movement the moment you lose the button.\nDon't use \"Break\" mode, which will cause step losses and other unexpected problem."
            n122 = event-data() -> ()  [unwired: 1 in, 8 out]
            n123 = local read "Motor hModule"() -> (w216:i32)
            n124 = call <userlib>:"mctl_SetMotionState.vi"("error in"=w218, "Motion State"=w215, "hModule In"=w216) -> ("error out"=w217:errorcluster)  [unwired: 1 in, 1 out]
          }
          event "Stop Motion": Mouse Up {
            w221 = u32 3 items=["Restart", "Stop", "Break", "Abort"] ("Motion State")
            # "Abort movement that is happening with no step losses"
            n125 = event-data() -> ()  [unwired: 1 in, 8 out]
            n126 = local read "Motor hModule"() -> (w220:i32)
            n127 = call <userlib>:"mctl_SetMotionState.vi"("Motion State"=w221, "hModule In"=w220) -> ("error out"=w219:errorcluster)  [unwired: 2 in, 1 out]
          }
          event "Reset Motion": Mouse Up {
            # "This function performs a reset of the machine control and the Motion Control DLL. The startup condition of the control is restored. A currently executed motion will be aborted immediately. Depending from the type of the connected control other, specific functions are executed. After calling the reset function, the machine resides in a \"Ready for operation\" state."
            n128 = event-data() -> ()  [unwired: 1 in, 8 out]
            n129 = local read "Motor hModule"() -> (w223:i32)
            n130 = call <userlib>:"mctl_Reset.vi"("hModule In"=w223) -> ("error out"=w222:errorcluster)  [unwired: 3 in, 1 out]
          }
          event "Reference": Mouse Up {
            # "The override is an additional velocity correction factor which is reckoned up with the current set velocities. \n\nThis function is used to set the override value of the Motion Control."
            # "Maybe move back to the zero point?"
            # "referrence run ?"
            # "set override"
            # "set vel"
            # "get vel"
            n131 = event-data() -> ()  [unwired: 1 in, 8 out]
            n132 = local read "Motor hModule"() -> (w233:i32)
            n133 = call <userlib>:"mctl_GetConfiguration.vi"("hModule In"=w233) -> ("error out"=w224:errorcluster, "Configuration"=w259:T17, "hModule Out"=w260:u32)  [unwired: 2 in]
            n134 = Unbundle By Name(w259) -> ("AxisConfig.AxisConfig 0.In Use"=w258:bool, "AxisConfig.AxisConfig 1.In Use"=w257:bool, "AxisConfig.AxisConfig 2.In Use"=w256:bool, "AxisConfig.AxisConfig 3.In Use"=w255:bool, "AxisConfig.AxisConfig 4.In Use"=w254:bool, "AxisConfig.AxisConfig 5.In Use"=w232:bool, "AxisConfig.AxisConfig 6.In Use"=w231:bool, "AxisConfig.AxisConfig 7.In Use"=w230:bool, "AxisConfig.AxisConfig 8.In Use"=w229:bool)
            n135 = local read "Manual Operation Control"() -> (w234:T1)
            n136 = Bundle("In Use"=w258, "In Use"=w257, "In Use"=w256, "In Use"=w255, "In Use"=w254, "In Use"=w232, "In Use"=w231, "In Use"=w230, "In Use"=w229) -> (w253:T18)  [unwired: 1 in]
            n137 = Unbundle By Name(w234) -> ("Speed Override (%)"=w239:dbl, "Linear.Speed"=w250:dbl, "Rotative.Speed"=w249:dbl)
            n138 = call <userlib>:"mctl_Reference.vi"("error in"=w224, "Reference Axis"=w253, "hModule In"=w260) -> ("error out"=w227:errorcluster, "hModule Out"=w238:u32)  [unwired: 1 in]
            n139 = Multiply(x=w250, y=1000.0) -> (x*y=w248:dbl)
            n140 = Multiply(x=w249, y=1296000.0) -> (x*y=w247:dbl)
            n141 = Multiply(x=75.0, y=1000.0) -> (x*y=w244:dbl)
            n142 = Multiply(x=2.8, y=1296000.0) -> (x*y=w243:dbl)
            n143 = call <userlib>:"mctl_GetVelocity.vi"("error in"=w227, "hModule In"=w238) -> ("error out"=w226:errorcluster, "Velocity"=w237:T15, "hModule Out"=w236:u32)  [unwired: 1 in]
            n144 = Bundle By Name(cluster=w237, "LiNormVel"=w248, "DrNormVel"=w247, "LiFastVel"=w244, "DrFastVel"=w243) -> (w240:T15)
            n145 = call <userlib>:"mctl_SetVelocity.vi"("error in"=w226, "Velocity"=w240, "hModule In"=w236) -> ("error out"=w225:errorcluster, "hModule Out"=w235:u32)  [unwired: 1 in]
            n146 = call <userlib>:"mctl_SetOverride.vi"("error in"=w225, "Override %"=w239, "hModule In"=w235) -> ("error out"=w228:errorcluster)  [unwired: 1 in, 1 out]
          }
          event "Leave HWLS": Mouse Up {
            # "leave Hardware Limit Switch \n\nAfter activating a hardware limit switch during a movement, the machine stops and the power supply of the machine is switched off for security reasons. If the hardware limit switch is still active after the machine has switched off, it is difficult to set the machine into an operative state."
            n147 = event-data() -> ()  [unwired: 1 in, 8 out]
            n148 = local read "Motor hModule"() -> (w268:i32)
            n149 = call <userlib>:"mctl_GetConfiguration.vi"("hModule In"=w268) -> ("error out"=w261:errorcluster, "Configuration"=w275:T17, "hModule Out"=w269:u32)  [unwired: 2 in]
            n150 = Unbundle By Name(w275) -> ("AxisConfig.AxisConfig 0.In Use"=w274:bool, "AxisConfig.AxisConfig 1.In Use"=w273:bool, "AxisConfig.AxisConfig 2.In Use"=w272:bool, "AxisConfig.AxisConfig 3.In Use"=w271:bool, "AxisConfig.AxisConfig 4.In Use"=w270:bool, "AxisConfig.AxisConfig 5.In Use"=w266:bool, "AxisConfig.AxisConfig 6.In Use"=w265:bool, "AxisConfig.AxisConfig 7.In Use"=w264:bool, "AxisConfig.AxisConfig 8.In Use"=w263:bool)
            n151 = Bundle("In Use"=w274, "In Use"=w273, "In Use"=w272, "In Use"=w271, "In Use"=w270, "In Use"=w266, "In Use"=w265, "In Use"=w264, "In Use"=w263) -> (w262:T18)  [unwired: 1 in]
            n152 = call <userlib>:"mctl_LeaveHWLS.vi"("error in"=w261, "Axis leave Limit"=w262, "hModule In"=w269) -> ("error out"=w267:errorcluster)  [unwired: 1 in, 1 out]
          }
          event "Test Mode": Mouse Up {
            # "Remarks \n\nNormally a Motion Control requires the execution of a reference run before it is fully operative. Since the reference run is not executed it is not possible to take access to the various movement functions of the Motion Control.\n \nIn some cases, e.g. during the start-up phase of working with a machine, it may be useful to access the movement functions without the previous execution of a reference run. The function mctl_SetTestMode() activates the so called \"Test mode\" which simulates a reference run if the complying function mctl_Reference() is called. //The current positions of each axis become the new machine zero point. //\n\nIn addition, the permanent checking of the hardware limit switches is switched off. The checking of hardware limit switches is used to set the Motion Control into an error state immediately after the activation of at least one hardware limit switch.// This feature enables you to move one or several axes into the mechanical stop for test purposes. //"
            n153 = event-data() -> ()  [unwired: 1 in, 8 out]
            n154 = local read "Motor hModule"() -> (w277:i32)
            n155 = call <userlib>:"mctl_GetStatus.vi"("hModule In"=w277) -> ("error out"=w278:errorcluster, "Status"=w282:T9, "hModule Out"=w279:u32)  [unwired: 2 in]
            n156 = Unbundle By Name(w282) -> ("Common.INTESTMODE"=w281:bool)
            n157 = Not(x=w281) -> (.not. x?=w280:bool)
            n158 = call <userlib>:"mctl_SetTestMode.vi"("error in"=w278, "Test Mode"=w280, "hModule In"=w279) -> ("error out"=w276:errorcluster)  [unwired: 1 in, 1 out]
          }
          event Mouse Down {
            n159 = event-data() -> ()  [unwired: 1 in, 8 out]
            n160 = flat-sequence {
              tunnel: ["Abs Position"] -> w286
              frame #0 {
                n161 = Wait (ms)(milliseconds to wait=u32 5) -> ()  [unwired: 1 out]
              }
              frame #1 {
              }
            }
            n162 = for {
              N: 1 -> [_]
              tunnel: w286 -> [w296]
              tunnel: [w309] -> w287
              tunnel: [w292] -> w283
              tunnel: w284 -> [w290]
              w303 = 1000
              n163 = Unbundle By Name(w296) -> ("OK Button"=w310:bool)
              n164 = Unbundle By Name(w296) -> ("Normal Move"=w293:bool, "Fast Move"=w295:bool, "Pos X"=w306:dbl, "Pos Y"=w305:dbl, "Pos Z"=w304:dbl, "Pos A"=w302:dbl)
              n165 = case shown="True" w310 {
                tunnel: w296 -> [w325 w331]
                tunnel: [w325 w326] -> w309
                frame False {
                }
                frame True {
                  n166 = local read "System Status"() -> (w332:T4)
                  n167 = Unbundle By Name(w332) -> ("Axis X.Position"=w330:dbl, "Axis Y.Position"=w329:dbl, "Axis Z.Position"=w328:dbl, "Axis A.Position"=w327:dbl)
                  n168 = Bundle By Name(cluster=w331, "Pos X"=w330, "Pos Y"=w329, "Pos Z"=w328, "Pos A"=w327) -> (w326:T3)
                }
              }
              n169 = local read "Motor hModule"() -> (w291:i32)
              n170 = Compound Arithmetic op=OR(w293, w295) -> (w294:bool)
              n171 = Multiply(x=w306, y=w303) -> (x*y=w300:dbl)
              n172 = Multiply(x=w305, y=w303) -> (x*y=w299:dbl)
              n173 = Multiply(x=w304, y=w303) -> (x*y=w298:dbl)
              n174 = Multiply(x=w302, y=1296000) -> (x*y=w297:dbl)
              n175 = Bundle By Name(cluster=T7 {"PosX"=0, "PosY"=0, "PosZ"=0, "PosA"=0, "PosB"=0, "PosC"=0, "PosU"=0, "PosV"=0, "PosW"=0} ("Abs"), "PosX"=w300, "PosY"=w299, "PosZ"=w298, "PosA"=w297) -> (w307:T7)
              n176 = case shown="True" w294 {
                tunnel: w307 -> [_ w316]
                tunnel: w293 -> [_ w315]
                tunnel: [w311 w314] -> w292
                tunnel: w291 -> [_ w313]
                tunnel: w290 -> [w311 w312]
                frame False {
                }
                frame True {
                  n177 = case shown="True" w315 {
                    tunnel: w316 -> [w320 w324]
                    tunnel: [w319 w323] -> w314
                    tunnel: w313 -> [w318 w322]
                    tunnel: w312 -> [w317 w321]
                    frame False {
                      n178 = call <userlib>:"mctl_FastAbs.vi"("error in"=w317, "FastAbs"=w320, "hModule In"=w318) -> ("error out"=w319:errorcluster)  [unwired: 1 in, 1 out]
                    }
                    frame True {
                      n179 = call <userlib>:"mctl_MoveAbs.vi"("error in"=w321, "Abs"=w324, "hModule In"=w322) -> ("error out"=w323:errorcluster)  [unwired: 1 in, 1 out]
                    }
                  }
                }
              }
            }
            n180 = local write "Abs Position"(w287) -> ()
          }
          event Mouse Down {
            n181 = event-data() -> ()  [unwired: 1 in, 8 out]
            n182 = flat-sequence {
              tunnel: ["Rel Position"] -> w336
              frame #0 {
                n183 = Wait (ms)(milliseconds to wait=u32 5) -> ()  [unwired: 1 out]
              }
              frame #1 {
              }
            }
            n184 = for {
              N: 1 -> [_]
              tunnel: w336 -> [w346]
              tunnel: [w359] -> w337
              tunnel: [w342] -> w333
              tunnel: w334 -> [w340]
              w353 = 1000
              n185 = Unbundle By Name(w346) -> ("OK Button"=w360:bool)
              n186 = Unbundle By Name(w346) -> ("Normal Move"=w343:bool, "Fast Move"=w345:bool, "Pos X"=w356:dbl, "Pos Y"=w355:dbl, "Pos Z"=w354:dbl, "Pos A"=w352:dbl)
              n187 = case shown="True" w360 {
                tunnel: w346 -> [w375 w381]
                tunnel: [w375 w376] -> w359
                frame False {
                }
                frame True {
                  n188 = local read "System Status"() -> (w382:T4)
                  n189 = Unbundle By Name(w382) -> ("Axis X.Position"=w380:dbl, "Axis Y.Position"=w379:dbl, "Axis Z.Position"=w378:dbl, "Axis A.Position"=w377:dbl)
                  n190 = Bundle By Name(cluster=w381, "Pos X"=w380, "Pos Y"=w379, "Pos Z"=w378, "Pos A"=w377) -> (w376:T3)
                }
              }
              n191 = local read "Motor hModule"() -> (w341:i32)
              n192 = Compound Arithmetic op=OR(w343, w345) -> (w344:bool)
              n193 = Multiply(x=w356, y=w353) -> (x*y=w350:dbl)
              n194 = Multiply(x=w355, y=w353) -> (x*y=w349:dbl)
              n195 = Multiply(x=w354, y=w353) -> (x*y=w348:dbl)
              n196 = Multiply(x=w352, y=1296000) -> (x*y=w347:dbl)
              n197 = Bundle By Name(cluster=T7 {"PosX"=0, "PosY"=0, "PosZ"=0, "PosA"=0, "PosB"=0, "PosC"=0, "PosU"=0, "PosV"=0, "PosW"=0} ("Abs"), "PosX"=w350, "PosY"=w349, "PosZ"=w348, "PosA"=w347) -> (w357:T7)
              n198 = case shown="True" w344 {
                tunnel: w357 -> [_ w366]
                tunnel: w343 -> [_ w365]
                tunnel: [w361 w364] -> w342
                tunnel: w341 -> [_ w363]
                tunnel: w340 -> [w361 w362]
                frame False {
                }
                frame True {
                  n199 = case shown="False" w365 {
                    tunnel: w366 -> [w370 w374]
                    tunnel: [w369 w373] -> w364
                    tunnel: w363 -> [w368 w372]
                    tunnel: w362 -> [w367 w371]
                    frame False {
                      n200 = call <userlib>:"mctl_FastRel.vi"("error in"=w367, "FastRel"=w370, "hModule In"=w368) -> ("error out"=w369:errorcluster)  [unwired: 1 in, 1 out]
                    }
                    frame True {
                      n201 = call <userlib>:"mctl_MoveRel.vi"("error in"=w371, "RelPOS"=w374, "hModule In"=w372) -> ("error out"=w373:errorcluster)  [unwired: 1 in, 1 out]
                    }
                  }
                }
              }
            }
            n202 = local write "Rel Position"(w337) -> ()
          }
          event Value Change {
            n203 = event-data() -> ()  [unwired: 1 in, 6 out]
            n204 = local read "Manual Operation Control"() -> (w385:T1)
            n205 = local read "Motor hModule"() -> (w383:i32)
            n206 = call <userlib>:"mctl_GetVelocity.vi"("hModule In"=w383) -> ("error out"=w390:errorcluster, "Velocity"=w389:T15, "hModule Out"=w391:u32)  [unwired: 2 in]
            n207 = Unbundle By Name(w385) -> ("Speed Override (%)"=w386:dbl, "Linear.Speed"=w396:dbl, "Rotative.Speed"=w395:dbl)
            n208 = Multiply(x=w396, y=1000.0) -> (x*y=w394:dbl)
            n209 = Multiply(x=w395, y=1296000.0) -> (x*y=w393:dbl)
            n210 = Bundle By Name(cluster=w389, "LiNormVel"=w394, "DrNormVel"=w393) -> (w392:T15)
            n211 = call <userlib>:"mctl_SetVelocity.vi"("error in"=w390, "Velocity"=w392, "hModule In"=w391) -> ("error out"=w387:errorcluster, "hModule Out"=w388:u32)  [unwired: 1 in]
            n212 = call <userlib>:"mctl_SetOverride.vi"("error in"=w387, "Override %"=w386, "hModule In"=w388) -> ("error out"=w384:errorcluster)  [unwired: 1 in, 1 out]
          }
        }
      }
    }
    frame #3 {
      w399 = FALSE ("Stop")
      # "Exit system"
      # "Restore value changes"
      # "Record current position information to position_zy.txt"
      # "Record current path information to path record.txt"
      n213 = local read "System Status"() -> (w404:T4)
      n214 = local read "Motor hModule"() -> (w405:i32)
      n215 = call <vilib>:"Application Directory.vi"() -> ("Application Directory"=w421:path)
      n216 = local read "MotionLibrary Path"() -> (w425:path)
      n217 = local read "MotionIni File In"() -> (w424:path)
      n218 = Unbundle By Name(w404) -> ("Initialized"=w403:bool)
      n219 = Bundle("MotionLibrary Path"=w425, "MotionIni File In"=w424) -> (w423:T8)  [unwired: 1 in]
      n220 = Build Path(base path=w421, name or relative path="path record.txt") -> (appended path=w430:path)
      n221 = Open/Create/Replace File(file path (use dialog)=w430, operation (0:open)=T5."replace or create") -> (refnum out=w429:refnum<file>, error out=w427:errorcluster)  [unwired: 4 in, 1 out]
      n222 = case shown="True" w403 {
        tunnel: w405 -> [_ w432]
        frame False {
        }
        frame True {
          n223 = call <userlib>:"mctl_Exit.vi"("hModule In"=w432) -> ()  [unwired: 3 in, 2 out]
        }
      }
      n224 = Write to Binary File(file (use dialog)=w429, data=w423, error in=w427, 5:FALSE ("prepend array or string size? (T)")) -> (refnum out=w428:refnum<file>, error out=w426:errorcluster)  [unwired: 2 in, 1 out]
      n225 = Close File(refnum=w428, error in=w426) -> ()  [unwired: 2 out]
      n226 = call <vilib>:"Application Directory.vi"() -> ("Application Directory"=w418:path)
      n227 = local read "Abs Position"() -> (w414:T3)
      n228 = local read "Rel Position"() -> (w415:T3)
      n229 = property on="Initialize" class="Bool (strict)"("BoolText.Text"="Initialize" ("Boolean Text.Text")) -> ()  [unwired: 2 in, 2 out]
      n230 = Bundle("Abs Position"=w414, "Rel Position"=w415) -> (w416:cluster{"Abs Position":T3, "Rel Position":T3})  [unwired: 1 in]
      n231 = Build Path(base path=w418, name or relative path="position_zy.txt") -> (appended path=w409:path)
      n232 = local write "Auto Run"(w399) -> ()
      n233 = local write "Exit"(w399) -> ()
      n234 = Open/Create/Replace File(file path (use dialog)=w409, operation (0:open)=T5."replace or create") -> (refnum out=w410:refnum<file>, error out=w412:errorcluster)  [unwired: 4 in, 1 out]
      n235 = Write to Binary File(file (use dialog)=w410, data=w416, error in=w412, 5:FALSE ("prepend array or string size? (T)")) -> (refnum out=w411:refnum<file>, error out=w413:errorcluster)  [unwired: 2 in, 1 out]
      n236 = Close File(refnum=w411, error in=w413) -> ()  [unwired: 2 out]
      n237 = local write "System Status"(T4 {"Axis X"={"Position"=0.0, "Limit NEG"=FALSE, "Limit  POS"=FALSE}, "Axis Y"={"Position"=0.0, "Limit NEG"=FALSE, "Limit  POS"=FALSE}, "Axis Z"={"Position"=0.0, "Limit NEG"=FALSE, "Limit  POS"=FALSE}, "Axis A"={"Position"=0.0, "Limit NEG"=FALSE, "Limit  POS"=FALSE}, "Initialized"=FALSE, " Moving"=FALSE, "Busy"=FALSE, "Need Ref."=FALSE, "Power Fail"=FALSE, "Test Mode"=FALSE, "Linear Speed"=0.0, "Rotativ Speed"=0.0, "Error Information"=""} ("System Status")) -> ()
      n238 = local read "Manual Operation Control"() -> (w402:T1)
      n239 = Bundle By Name(cluster=w402, "Axis-A Movement"=FALSE) -> (w400:T1)
      n240 = local write "Manual Operation Control"(w400) -> ()
    }
  }
